vi "Day 21 - Monkey Math.vi"() -> ()   [LabVIEW 2020, in "AoC 2022.lvlib"]
uses:
  AoC 2022.lvlib
  <vilib>/Utility/miscctls.llb/LVMapReplaceAction.ctl
panel:
  in  "Puzzle Input":string="root: pppw + sjmn\ndbpl: 5\ncczh: sllz + lgvd\nzczc: 2\nptdq: humn - dvpt\ndvpt: 3\nlfqf: 4\nhumn: 5\nljgn: 2\nsjmn: drzm * dbpl\nsllz: 4\npppw: cczh / lfqf\nlgvd: ljgn * ptdq\ndrzm: hmdt - zczc\nhmdt: 32"
  out "Puzzle Part-2 Answer":string
  out "Puzzle Answer":string
  # "Press Ctrl+M & Enter the Puzzle Input and run the VI"
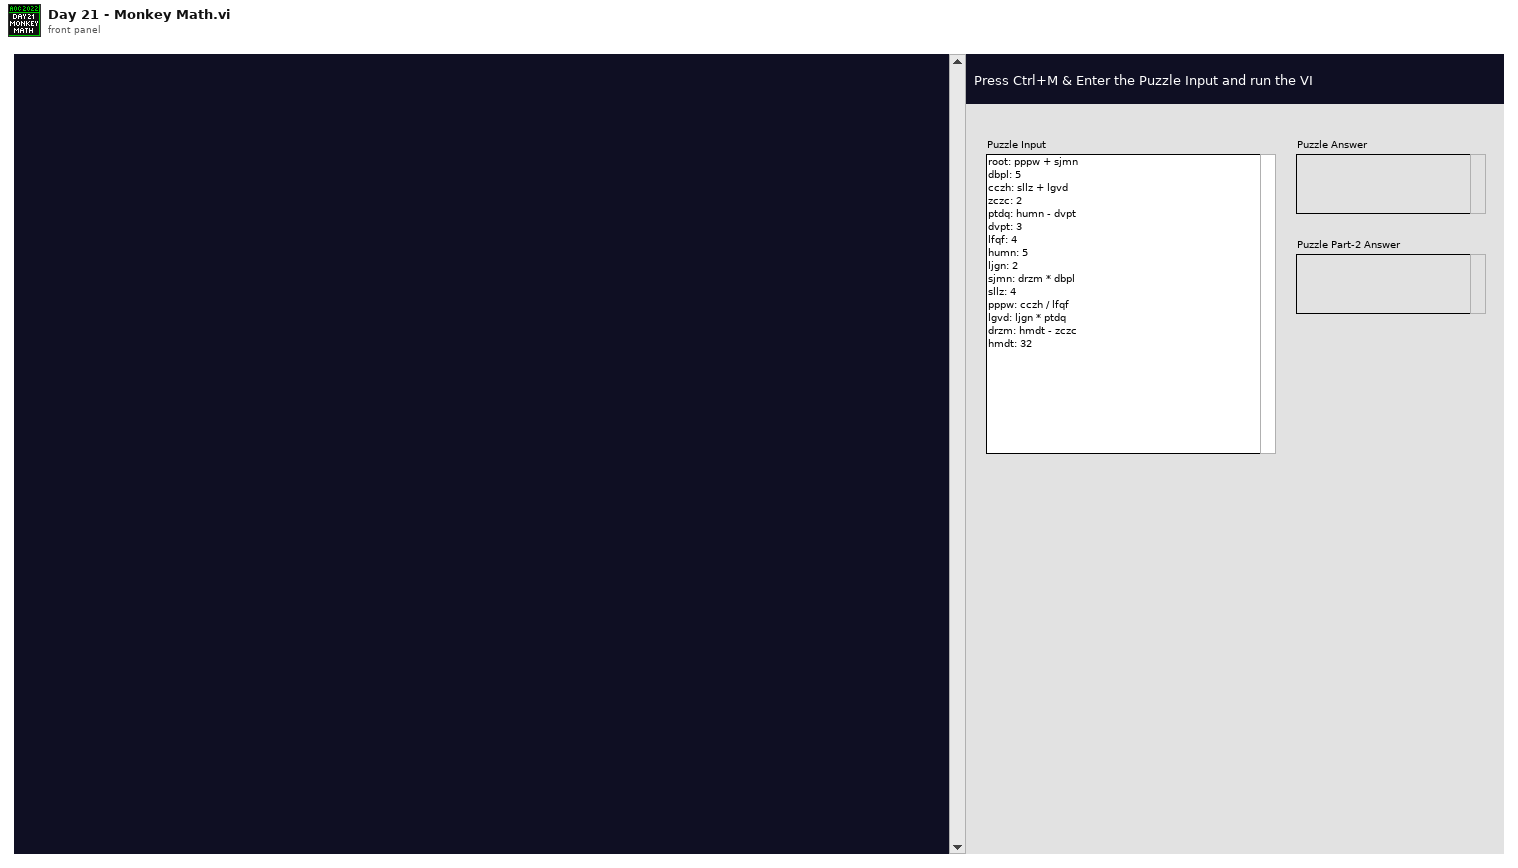
[diagram p1: front panel]
types:
  T1 = typedef "LVMapReplaceAction.ctl" = enum32{"Modify Entry only if found", "Add or Modify Entry", "Delete Entry"}
  T2 = typedef "AoC 2022.lvlib/Monkeys.ctl" = map{string, T3}
  T3 = typedef "AoC 2022.lvlib/Monkey.ctl" = cluster{"Items":u64[], "Bored Operation":string, "Inspection Operation":string, "Test: Divisible By":u64, "Test: True - Monkey":string, "Test: False - Monkey":string, "#Inspected":i32}
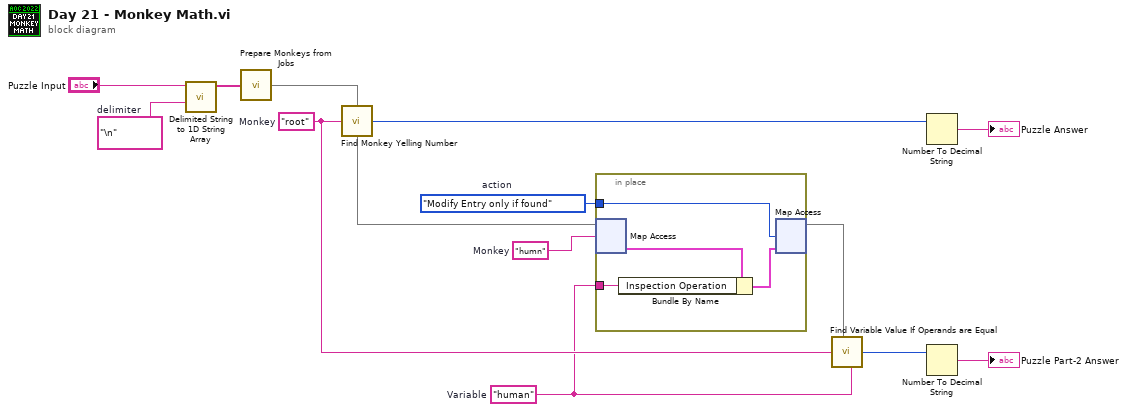
[diagram p0: block diagram]
diagram:
  w1 = "human"  # Variable
  w4 = LVMapReplaceAction."Modify Entry only if found"  # action
  w5 = "humn"  # Monkey
  w7 = "root"  # Monkey
  w11 = "\n"  # delimiter
  n1 = call <vilib>:"Delimited String to 1D String Array.vi"("delimiter"=w11, "delimited string"="Puzzle Input") -> ("string array"=w10:string[])  [unwired: 9 in]
  n2 = call "Prepare Monkeys from Jobs.vi"("Monkey Jobs"=w10) -> ("Monkeys"=w6:T2)  [unwired: 2 in]
  n3 = call "Find Monkey Yelling Number.vi"("Monkey"=w7, "Monkeys"=w6) -> ("Monkey Yelling Number"=w8:u64)
  n4 = in-place {
    in-place-border: w4 -> [w17]
    in-place-border: w1 -> [w14]
    n5 = in-place-map #1(w6, w5) -> (w16:T3)  [unwired: 1 in, 1 out]
    n6 = Bundle By Name(cluster=w16, "Inspection Operation"=w14) -> (w15:T3)
    n7 = in-place-map #1(w15, w17) -> (w3:T2)  [unwired: 2 out]
  }
  n8 = call "Find Variable Value If Operands are Equal.vi"("Monkey"=w7, "Monkeys"=w3, "Variable"=w1) -> ("Variable Value"=w2:u64)
  n9 = Number To Decimal String(number=w8) -> (decimal integer string=→"Puzzle Answer":string)  [unwired: 1 in]
  n10 = Number To Decimal String(number=w2) -> (decimal integer string=→"Puzzle Part-2 Answer":string)  [unwired: 1 in]
